vi "测试-生成excel报表.vi"() -> ()   [LabVIEW 2018]
panel:
  in  "表格控件":string[][](table)
  in  "测试人":string
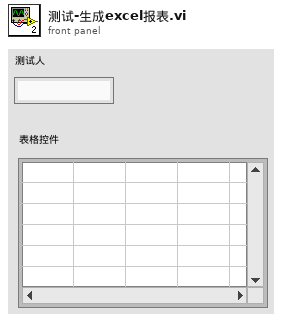
[diagram p1: front panel]
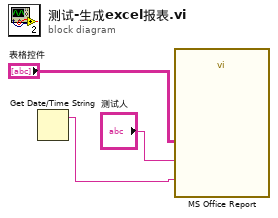
[diagram p0: block diagram]
diagram:
  n1 = Get Date/Time String() -> (date string=w3:string)  [unwired: 3 in, 1 out]
  n2 = call "MS Office Report"("data"="表格控件", "name"="测试人", "time"=w3) -> ()  [unwired: 24 in, 1 out]
